vi "FPGA_controller.vi"() -> ()   [LabVIEW 2017]
uses:
  <vilib>/rvi/Emulation/niFpgaGetClockAttributes.vi
  <vilib>/rvi/Emulation/niFpgaSctlEmulationGetInTimedLoop.vi
  <vilib>/rvi/Emulation/niFpgaEmulationReportErrorSimple.vi
  <vilib>/rvi/eio/common/nirviEmuTemplateMethod_errors.vi
  <vilib>/rvi/Emulation/niFpgaCriticalErrorInLSC.vi
  <vilib>/eio/EIONode/EIONode.xnode
panel:
  in  "Input_6":bool
  in  "Input_5":bool
  in  "Input_4":bool
  in  "Input_3":bool
  in  "Input_2":bool
  in  "Input_1":bool
  out "Translated":i16
  out "VALID":bool
  in  "m_first u2":fxp<+/-,64,32>=-0.8999999999068677 format="%#_42g"
  in  "m_first u1":fxp<+/-,64,32>=-0.8999999999068677 format="%#_42g"
  in  "Scale u2":fxp<+/-,64,42>=5.0 format="%#_35g"
  in  "Offset u2":fxp<+/-,64,41>=2.0 format="%#_36g"
  in  "Scale u1":fxp<+/-,64,42>=5.0 format="%#_35g"
  in  "Offset u1":fxp<+/-,64,41>=2.0 format="%#_36g"
  in  "eta u":fxp<+,16,1>=0.29998779296875 format="%#_42g"
  in  "Scale x2":fxp<+/-,32,16>=10.0 format="%#_21g"
  in  "m_first x2":fxp<+/-,49,33> format="%#_26g"
  in  "Offset x2":fxp<+/-,48,32> format="%#_26g"
  in  "Offset x3":fxp<+/-,48,32>=5.0 format="%#_26g"
  in  "m_first x3":fxp<+/-,32,16>=-3.399993896484375 format="%#_21g"
  in  "Scale x3":fxp<+/-,32,16>=10.0 format="%#_21g"
  in  "1/eta x":fxp<+,3,3>=5.0 format="%#_21g"
  in  "m_first x1":fxp<+/-,49,33> format="%#_26g"
  in  "Offset x1":fxp<+/-,48,32> format="%#_26g"
  in  "Scale x1":fxp<+/-,32,16>=10.0 format="%#_21g"
  in  "stop":bool
  # "INPUTS CONVERSION"
  # "STATES CONVERSION"
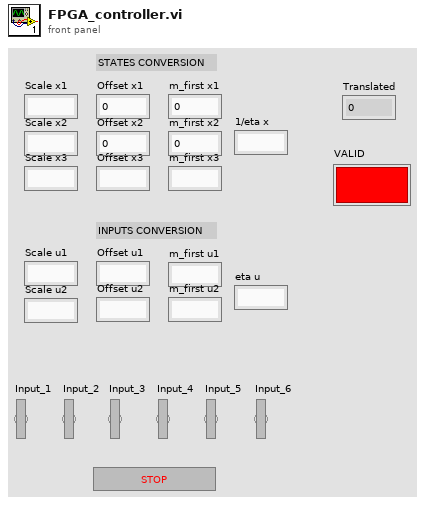
[diagram p1: front panel]
types:
  T1 = cluster{"Boolean array[0]":bool, "Boolean array[1]":bool, "Boolean array[2]":bool, "Boolean array[3]":bool, "Boolean array[4]":bool, "Boolean array[5]":bool, "Boolean array[6]":bool, "Boolean array[7]":bool, "Boolean array[8]":bool, "Boolean array[9]":bool, "Boolean array[10]":bool, "Boolean array[11]":bool, "Boolean array[12]":bool, "Boolean array[13]":bool, "Boolean array[14]":bool, "Boolean array[15]":bool, "Boolean array[16]":bool, "Boolean array[17]":bool}
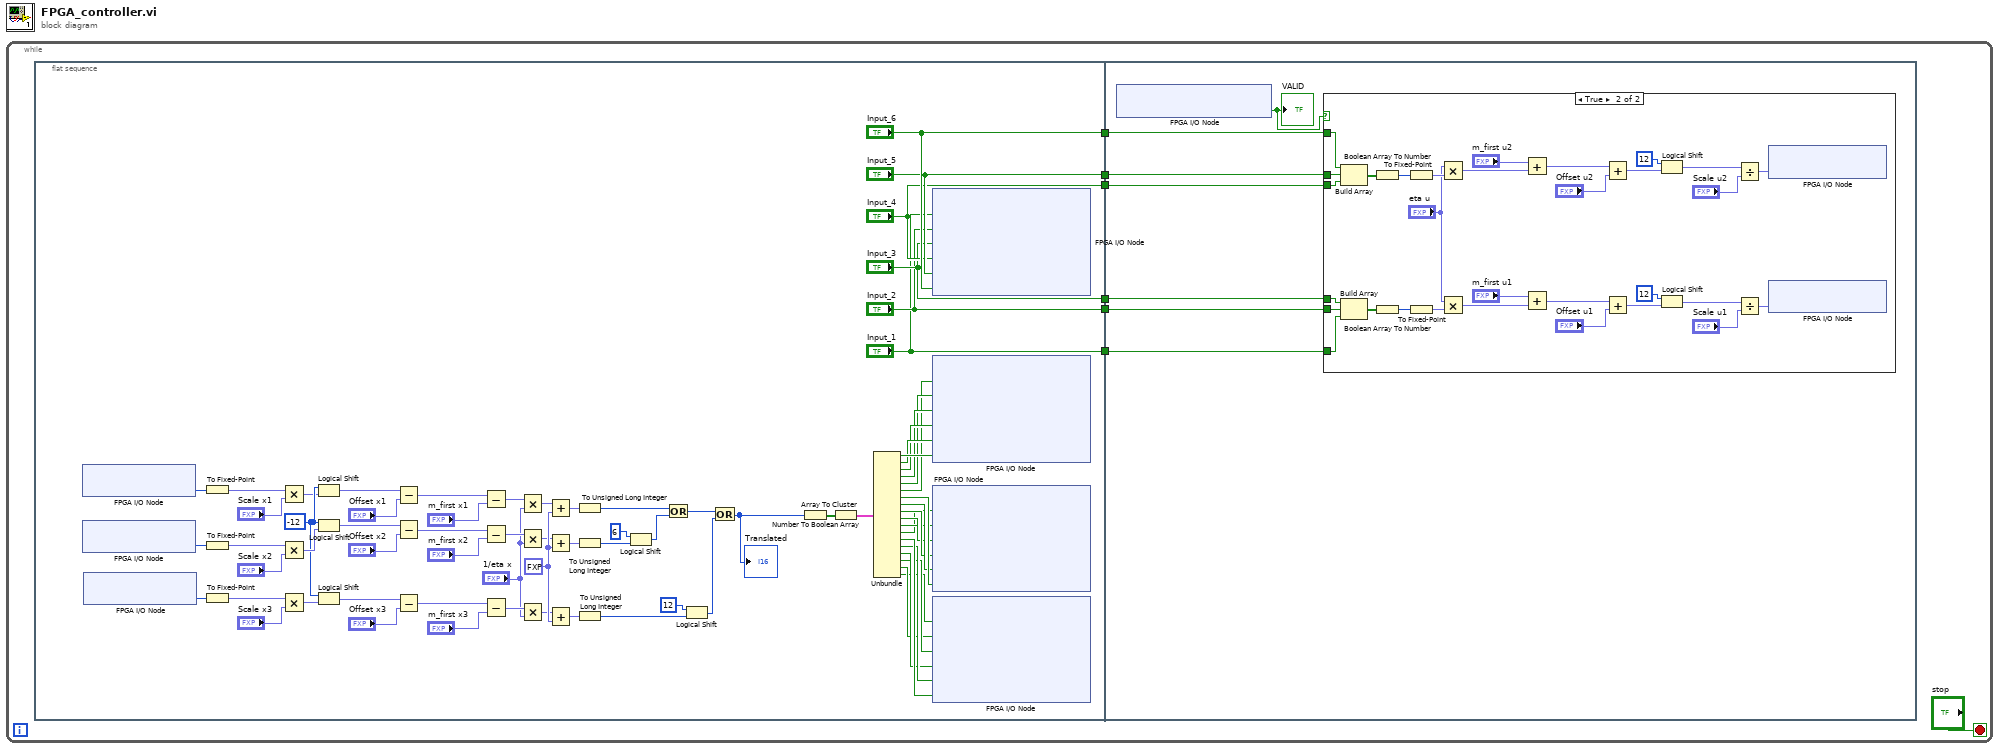
[diagram p0: block diagram]
diagram:
  n1 = while {
    stop <- "stop" stop-if-true
    n2 = flat-sequence {
      tunnel: ["Input_1"] -> w6
      tunnel: ["Input_2"] -> w5
      tunnel: ["Input_3"] -> w4
      tunnel: ["Input_4"] -> w3
      tunnel: ["Input_5"] -> w2
      tunnel: ["Input_6"] -> w1
      tunnel: w6 -> [w85]
      tunnel: w5 -> [w84]
      tunnel: w4 -> [w83]
      tunnel: w3 -> [w82]
      tunnel: w2 -> [w81]
      tunnel: w1 -> [w80]
      frame #0 {
        w48 = fxp<+,2,1> 0.5 ("y")
        w43 = i16 -12 ("y")
        n3 = xnode "FPGA I/O Node"() -> ("ConnectorA/AI0"=w13:u16)  [unwired: 1 in, 1 out]
        n4 = xnode "FPGA I/O Node"() -> ("ConnectorA/AI1"=w11:u16)  [unwired: 1 in, 1 out]
        n5 = xnode "FPGA I/O Node"() -> ("ConnectorB/AI0"=w9:u16)  [unwired: 1 in, 1 out]
        n6 = To Fixed-Point(number=w13) -> (fixed-point=w12:fxp<+,16,16>)  [unwired: 1 in]
        n7 = To Fixed-Point(number=w11) -> (fixed-point=w10:fxp<+,16,16>)  [unwired: 1 in]
        n8 = To Fixed-Point(number=w9) -> (fixed-point=w8:fxp<+,16,16>)  [unwired: 1 in]
        n9 = Multiply(x=w12, y="Scale x1") -> (x*y=w39:fxp<+/-,48,32>)
        n10 = Multiply(x=w10, y="Scale x2") -> (x*y=w49:fxp<+/-,48,32>)
        n11 = Multiply(x=w8, y="Scale x3") -> (x*y=w41:fxp<+/-,48,32>)
        n12 = Logical Shift(y=w43, x=w39) -> (x << y=w36:fxp<+/-,48,32>)
        n13 = Logical Shift(y=w43, x=w49) -> (x << y=w33:fxp<+/-,48,32>)
        n14 = Logical Shift(y=w43, x=w41) -> (x << y=w40:fxp<+/-,48,32>)
        n15 = Subtract(x=w36, y="Offset x1") -> (x-y=w37:fxp<+/-,49,33>)
        n16 = Subtract(x=w33, y="Offset x2") -> (x-y=w34:fxp<+/-,49,33>)
        n17 = Subtract(x=w40, y="Offset x3") -> (x-y=w42:fxp<+/-,49,33>)
        n18 = Subtract(x=w37, y="m_first x1") -> (x-y=w38:fxp<+/-,50,34>)
        n19 = Subtract(x=w34, y="m_first x2") -> (x-y=w32:fxp<+/-,50,34>)
        n20 = Subtract(x=w42, y="m_first x3") -> (x-y=w45:fxp<+/-,50,34>)
        n21 = Multiply(x=w38, y="1/eta x") -> (x*y=w35:fxp<+/-,53,37>)
        n22 = Multiply(x=w32, y="1/eta x") -> (x*y=w31:fxp<+/-,53,37>)
        n23 = Multiply(x=w45, y="1/eta x") -> (x*y=w44:fxp<+/-,52,36>)
        n24 = Add(x=w35, y=w48) -> (x+y=w58:fxp<+/-,53,37>)
        n25 = Add(x=w31, y=w48) -> (x+y=w47:fxp<+/-,53,37>)
        n26 = Add(x=w44, y=w48) -> (x+y=w46:fxp<+/-,52,36>)
        n27 = To Unsigned Long Integer(number=w58) -> (unsigned 32bit integer=w54:u32)
        n28 = To Unsigned Long Integer(number=w47) -> (unsigned 32bit integer=w56:u32)
        n29 = To Unsigned Long Integer(number=w46) -> (unsigned 32bit integer=w52:u32)
        n30 = Logical Shift(y=6, x=w56) -> (x << y=w55:u32)
        n31 = Or(x=w54, y=w55) -> (x .or. y?=w50:u32)
        n32 = Logical Shift(y=12, x=w52) -> (x << y=w51:u32)
        n33 = Or(x=w50, y=w51) -> (x .or. y?=w20:u32)
        "Translated" <- w20
        n34 = Number To Boolean Array(number=w20) -> (Boolean array=w59:bool[])
        n35 = Array To Cluster(array=w59) -> (cluster=w78:T1)
        n36 = Unbundle(w78) -> ("Boolean array[0]"=w77:bool, "Boolean array[1]"=w76:bool, "Boolean array[2]"=w75:bool, "Boolean array[3]"=w74:bool, "Boolean array[4]"=w73:bool, "Boolean array[5]"=w72:bool, "Boolean array[6]"=w71:bool, "Boolean array[7]"=w70:bool, "Boolean array[8]"=w69:bool, "Boolean array[9]"=w68:bool, "Boolean array[10]"=w67:bool, "Boolean array[11]"=w66:bool, "Boolean array[12]"=w65:bool, "Boolean array[13]"=w64:bool, "Boolean array[14]"=w63:bool, "Boolean array[15]"=w62:bool, "Boolean array[16]"=w61:bool, "Boolean array[17]"=w60:bool)
        n37 = xnode "FPGA I/O Node"("Component-Level IP\\pi18"="Input_1", "Component-Level IP\\pi19"="Input_2", "Component-Level IP\\pi20"="Input_3", "Component-Level IP\\pi21"="Input_4", "Component-Level IP\\pi22"="Input_5", "Component-Level IP\\pi23"="Input_6") -> ()  [unwired: 6 in, 6 out]
        n38 = xnode "FPGA I/O Node"("Component-Level IP\\pi00"=w72, "Component-Level IP\\pi01"=w73, "Component-Level IP\\pi02"=w74, "Component-Level IP\\pi03"=w75, "Component-Level IP\\pi04"=w76, "Component-Level IP\\pi05"=w77) -> ()  [unwired: 6 in, 6 out]
        n39 = xnode "FPGA I/O Node"("Component-Level IP\\pi06"=w66, "Component-Level IP\\pi07"=w67, "Component-Level IP\\pi08"=w68, "Component-Level IP\\pi09"=w69, "Component-Level IP\\pi10"=w70, "Component-Level IP\\pi11"=w71) -> ()  [unwired: 6 in, 6 out]
        n40 = xnode "FPGA I/O Node"("Component-Level IP\\pi12"=w60, "Component-Level IP\\pi13"=w61, "Component-Level IP\\pi14"=w62, "Component-Level IP\\pi15"=w63, "Component-Level IP\\pi16"=w64, "Component-Level IP\\pi17"=w65) -> ()  [unwired: 6 in, 6 out]
      }
      frame #1 {
        n41 = xnode "FPGA I/O Node"() -> ("Component-Level IP\\po0"=w79:bool)  [unwired: 1 in, 1 out]
        "VALID" <- w79
        n42 = case shown="True" w79 {
          tunnel: w85 -> [_ w98]
          tunnel: w84 -> [_ w97]
          tunnel: w83 -> [_ w96]
          tunnel: w82 -> [_ w95]
          tunnel: w81 -> [_ w94]
          tunnel: w80 -> [_ w93]
          frame False {
          }
          frame True {
            n43 = Build Array(w93, w94, w95) -> (w106:bool[])
            n44 = Build Array(w96, w97, w98) -> (w115:bool[])
            n45 = Boolean Array To Number(Boolean array=w106) -> (number=w104:u8)
            n46 = Boolean Array To Number(Boolean array=w115) -> (number=w113:u8)
            n47 = To Fixed-Point(number=w104) -> (fixed-point=w103:fxp<+,8,8>)  [unwired: 1 in]
            n48 = To Fixed-Point(number=w113) -> (fixed-point=w112:fxp<+,8,8>)  [unwired: 1 in]
            n49 = Multiply(x="eta u", y=w103) -> (x*y=w107:fxp<+,24,9>)
            n50 = Multiply(x="eta u", y=w112) -> (x*y=w116:fxp<+,24,9>)
            n51 = Add(x="m_first u2", y=w107) -> (x+y=w105:fxp<+/-,64,33>)
            n52 = Add(x="m_first u1", y=w116) -> (x+y=w114:fxp<+/-,64,33>)
            n53 = Add(x=w105, y="Offset u2") -> (x+y=w102:fxp<+/-,64,42>)
            n54 = Add(x=w114, y="Offset u1") -> (x+y=w111:fxp<+/-,64,42>)
            n55 = Logical Shift(y=i16 12, x=w102) -> (x << y=w100:fxp<+/-,64,42>)
            n56 = Logical Shift(y=i16 12, x=w111) -> (x << y=w109:fxp<+/-,64,42>)
            n57 = Divide(x=w100, y="Scale u2") -> (x/y=w99:fxp<+/-,64,65>)
            n58 = Divide(x=w109, y="Scale u1") -> (x/y=w108:fxp<+/-,64,65>)
            n59 = xnode "FPGA I/O Node"("ConnectorB/AO1"=w99) -> ()  [unwired: 1 in, 1 out]
            n60 = xnode "FPGA I/O Node"("ConnectorB/AO0"=w108) -> ()  [unwired: 1 in, 1 out]
          }
        }
      }
    }
  }
